vi "temporary CE GUI main.vi"() -> ()   [LabVIEW 2020]
uses:
  General AC source/Type definitions/AC Source.ctl
  General AC source/Type definitions/AC Source type.ctl
  General DC meter/Type definitions/DC meter.ctl
  General DC meter/Type definitions/DC meter type.ctl
  FR Measurement/Type definitions/FR Measuement properties.ctl
  FR Utilities/Type definitions/FR Template definition.ctl
panel:
  out "Array":i32[](array[numeric])
  in  "Numeric":i32=100
  out "freq / PFI0 A / PFI0 unc(A) / PFI1 A / PFI0 unc(A)":string[][](array[string])
  out "error out":errorcluster
  in  "Skip waiting":bool caption="Abort"
  in  "Abort":bool
  in  "TWM status":string
  in  "mesurement status":string
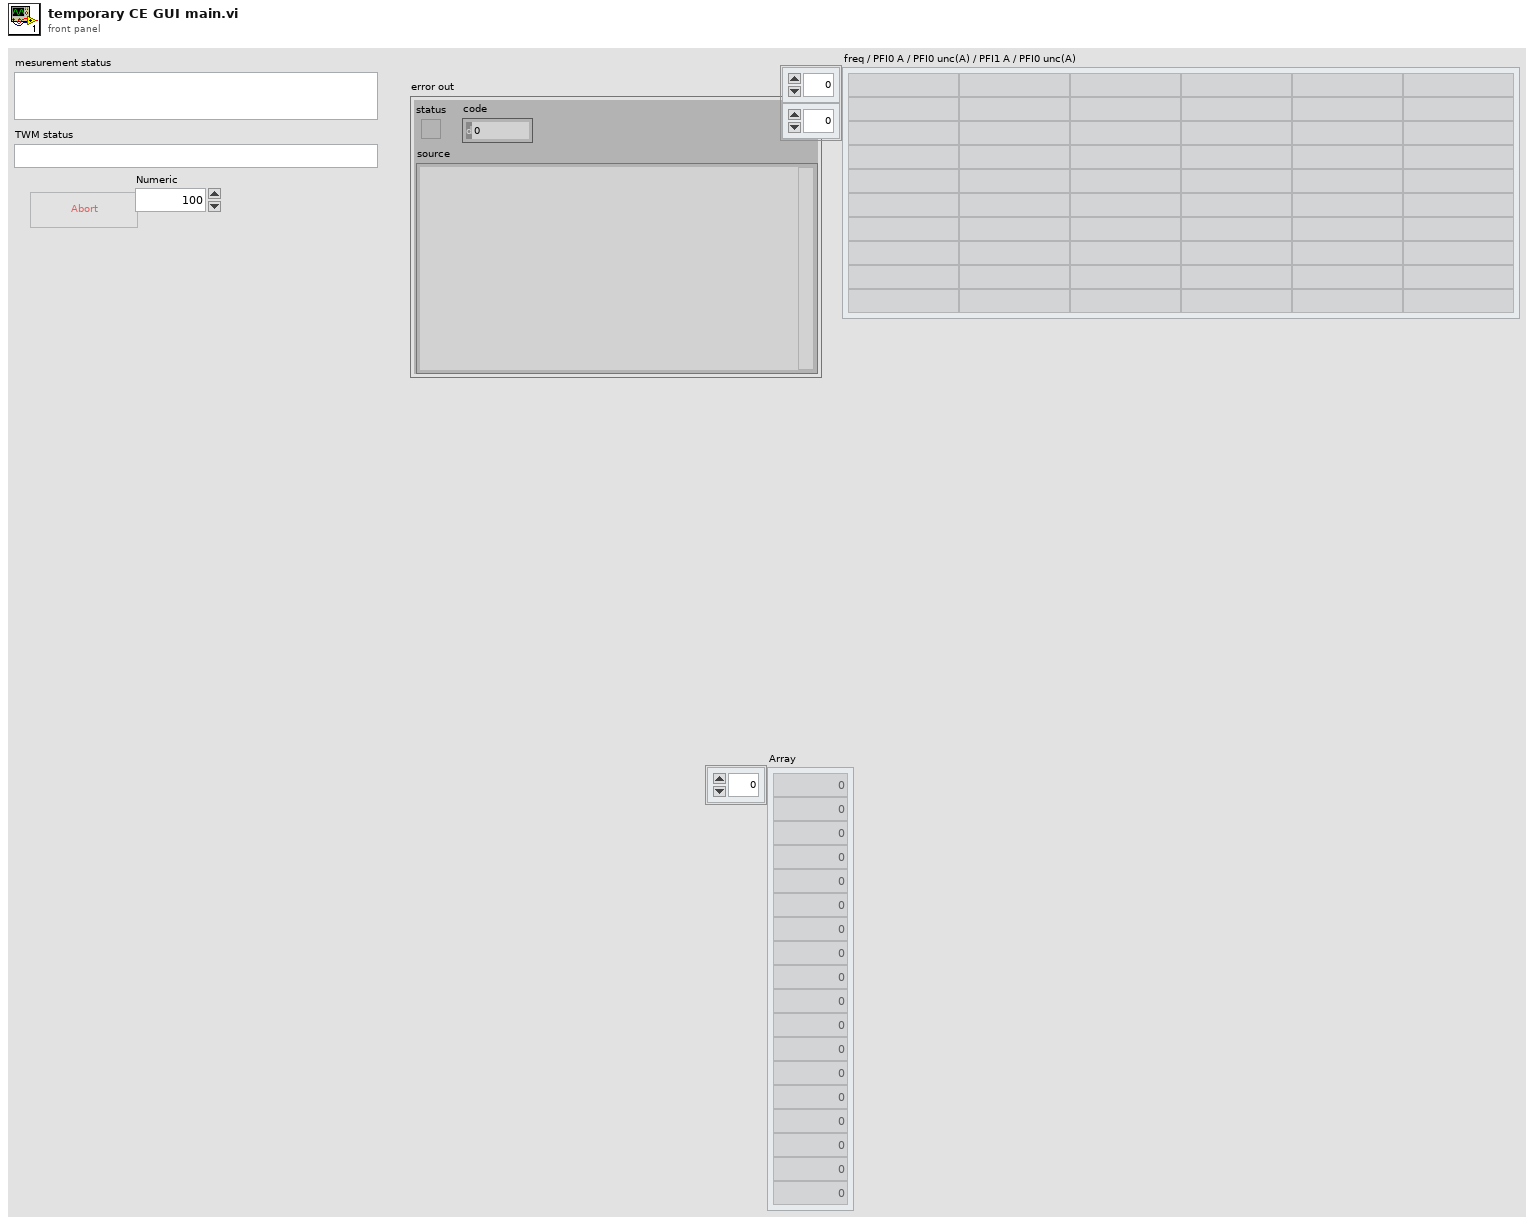
[diagram p1: front panel]
types:
  T1 = typedef "AC Source type.ctl" = enum16{"Fluke 5XXX calibrator", "Tektronix AFG3000 series", "dummy"}
  T2 = typedef "AC Source.ctl" = cluster{"AC Source type":T1, "VISA":refnum<visa-resource-name>, "Ref. clock (Hz)":dbl, "status ref":refnum<vi>}
  T3 = typedef "DC meter.ctl" = cluster{"DC meter type":T4, "DC meter VISA":refnum<visa-resource-name>, "NPLC":i32, "status ref":refnum<vi>}
  T4 = typedef "DC meter type.ctl" = enum16{"H/A/K 3458", "FLuke 8508A", "dummy"}
  T5 = typedef "FR Measuement properties.ctl" = cluster{"Measurement frequencies (Hz)":dbl[], "Sampling frequency (Hz)":dbl, "Signal amplitude (V)":dbl, "AC-DC settle time (s)":dbl, "Record length (multiples of period)":dbl[], "Measurement template file":path, "Row of START keyword":i32, "Row of STOP keyword":i32, "Calculate RMS from samples":bool, "AC-DC warm up time (s)":dbl, "Measurement template line":i32[], "DC meter readings No.":i32, "Algorithm":string}
  T6 = typedef "FR Template definition.ctl" = cluster{"Keywords column":i32, "Sig. freq. column":i32, "Rec. len. column":i32, "Meas. points. row min to read":i32, "Meas. points. row max to read":i32, "Properties column":i32, "Properties row start":i32, "Properties row end":i32, "Keyword START regexp":string, "Keyword STOP regexp":string, "HW data column":i32, "HW data row start":i32, "HW data row end":i32, "TIme and date column start":i32, "Digitizer value column start ":i32, "DC mean column start ":i32, "DC readings column start":i32}
  T7 = cluster{"AC Source":T2, "TWM pipe":string, "Measurement status ref":refnum<vi>, "TWM Status ref":refnum<vi>, "Abort ref":refnum<vi>, "DC meter":T3, "Measurement properties":T5, "Skip waiting ref":refnum<vi>, "Octave paths":cluster{"GNU Octave path":path, "TWM+QWTB path":path, "lvlib path":path}, "Template definition":T6}
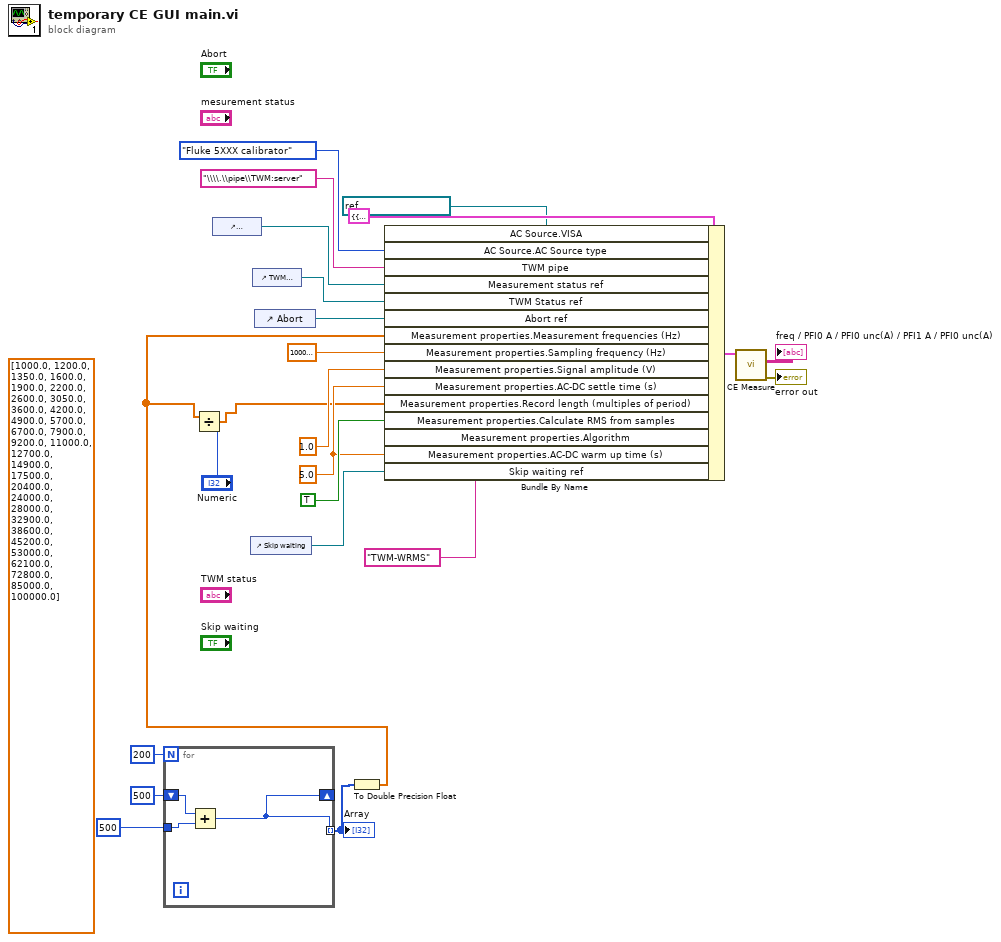
[diagram p0: block diagram]
diagram:
  w13 = 5.0 ("Measurement properties.AC-DC settle time (s)")
  (unwired) dbl[] [1000.0, 1200.0, 1350.0, 1600.0, 1900.0, 2200.0, 2600.0, 3050.0, 3600.0, 4200.0, 4900.0, 5700.0, 6700.0, 7900.0, 9200.0, 11000.0, 12700.0, 14900.0, 17500.0, 20400.0, 24000.0, 28000.0, 32900.0, 38600.0, 45200.0, 53000.0, 62100.0, 72800.0, 85000.0, 100000.0] ("Measurement properties.Measurement frequencies (Hz)")
  n1 = for {
    N: 200 -> [_]
    tunnel: 500 ("Numeric") -> [w26]
    shift-right: [w24] -> _
    shift-left: 500 -> [w25]
    tunnel: [w24] -> w2 mode=indexing
    n2 = Add(x=w25, y=w26) -> (x+y=w24:i32)
  }
  "Array" <- w2
  n3 = control-ref of="mesurement status"() -> (w19:refnum<vi>)
  n4 = control-ref of="Skip waiting"() -> (w12:refnum<vi>)
  n5 = control-ref of="TWM status"() -> (w18:refnum<vi>)
  n6 = control-ref of="Abort"() -> (w17:refnum<vi>)
  n7 = To Double Precision Float(number=w2) -> (double precision float=w1:dbl[])
  n8 = Divide(x=w1, y="Numeric") -> (x/y=w6:dbl[])
  n9 = Bundle By Name(cluster=T7 {"AC Source"={"AC Source type"=enum."dummy", "VISA"="", "Ref. clock (Hz)"=0.0, "status ref"=refnum}, "TWM pipe"="\\\\.\\pipe\\TWM:server", "Measurement status ref"=refnum, "TWM Status ref"=refnum, "Abort ref"=refnum, "DC meter"={"DC meter type"=enum."H/A/K 3458", "DC meter VISA"="", "NPLC"=10, "status ref"=refnum}, "Measurement properties"={"Measurement frequencies (Hz)"=[1000.0, 2000.0], "Sampling frequency (Hz)"=500000.0, "Signal amplitude (V)"=4.5, "AC-DC settle time (s)"=1.0, "Record length (multiples of period)"=[1000.0, 2000.0], "Measurement template file"=path "d:/mereni/smazat2/smazat2", "Row of START keyword"=1, "Row of STOP keyword"=0, "Calculate RMS from samples"=FALSE, "AC-DC warm up time (s)"=1.0, "Measurement template line"=[10, 20], "DC meter readings No."=10, "Algorithm"="TWM-WFFT"}, "Skip waiting ref"=refnum, "Octave paths"={"GNU Octave path"=path "C:/Program Files/GNU Octave/Octave-6.2.0/mingw64/bin", "TWM+QWTB path"=path "C:/Users/labina/Desktop/TWM-1.8.7.0-full/octprog", "lvlib path"=path "D:/martin/WAC/WACsw - github/control_software/Filter function meter/external libraries/GOLPI 0.7.3.1 source distribution LV 20.0 32 bit/lv_proc.dll"}, "Template definition"={"Keywords column"=0, "Sig. freq. column"=1, "Rec. len. column"=2, "Meas. points. row min to read"=9, "Meas. points. row max to read"=1509, "Properties column"=4, "Properties row start"=1, "Properties row end"=5, "Keyword START regexp"="", "Keyword STOP regexp"="", "HW data column"=7, "HW data row start"=1, "HW data row end"=3, "TIme and date column start"=3, "Digitizer value column start "=4, "DC mean column start "=6, "DC readings column start"=10}} ("CEmeter settings"), "AC Source.VISA"=refnum<visa-resource-name> "GPIB0::5::INSTR", "AC Source.AC Source type"=AC_Source_type."Fluke 5XXX calibrator", "TWM pipe"="\\\\.\\pipe\\TWM:server", "Measurement status ref"=w19, "TWM Status ref"=w18, "Abort ref"=w17, "Measurement properties.Measurement frequencies (Hz)"=w1, "Measurement properties.Sampling frequency (Hz)"=10000000.0, "Measurement properties.Signal amplitude (V)"=1.0, "Measurement properties.AC-DC settle time (s)"=w13, "Measurement properties.Record length (multiples of period)"=w6, "Measurement properties.Calculate RMS from samples"=TRUE, "Measurement properties.Algorithm"="TWM-WRMS", "Measurement properties.AC-DC warm up time (s)"=w13, "Skip waiting ref"=w12) -> (w22:T7)
  n10 = call "CE Measure.vi"("CEmeter settings"=w22) -> ("error out"=→"error out":errorcluster, "TWM result as string"=→"freq / PFI0 A / PFI0 unc(A) / PFI1 A / PFI0 unc(A)":string[][])  [unwired: 9 in]
